vi "Handle Valve Status.vi"(10 "Response Data":T1, 11 "Control Valves in":T2) -> (3 "Control Valves out":T2)   [LabVIEW 2024, in "pumploop_client.lvlib"]
uses:
  pumploop_client/pumploop_client.lvlib
  controls/Valves--cluster.ctl
  pumploop_client/RPC Messages/pumploop_Valves.ctl
panel:
  # "Open"
  # "Closed"
  # "Open"
  # "Closed"
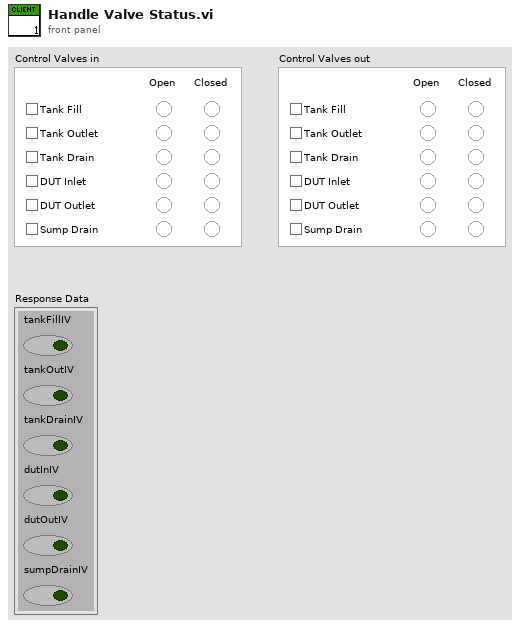
[diagram p1: front panel]
types:
  T1 = typedef "pumploop_client.lvlib/pumploop_Valves.ctl" = cluster{"tankFillIV":bool, "tankOutIV":bool, "tankDrainIV":bool, "dutInIV":bool, "dutOutIV":bool, "sumpDrainIV":bool}
  T2 = typedef "Valves--cluster.ctl" = cluster{"Tank Fill":bool, "Tank Outlet":bool, "Tank Drain":bool, "DUT Inlet":bool, "DUT Outlet":bool, "Sump Drain":bool, "Tank Fill Open":bool, "Tank Fill Closed":bool, "Tank Outlet Open":bool, "Tank Outlet Closed":bool, "Tank Drain Open":bool, "Tank Drain Closed":bool, "DUT Inlet Open":bool, "DUT Inlet Closed":bool, "DUT Outlet Open":bool, "DUT Outlet Closed":bool, "Sump Drain Open":bool, "Sump Drain Closed":bool}
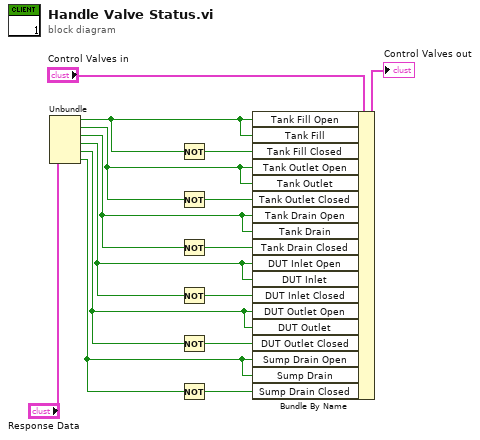
[diagram p0: block diagram]
diagram:
  n1 = Unbundle("Response Data") -> ("tankFillIV"=w6:bool, "tankOutIV"=w5:bool, "tankDrainIV"=w4:bool, "dutInIV"=w3:bool, "dutOutIV"=w2:bool, "sumpDrainIV"=w1:bool)
  n2 = Not(x=w6) -> (.not. x?=w8:bool)
  n3 = Not(x=w5) -> (.not. x?=w9:bool)
  n4 = Not(x=w4) -> (.not. x?=w10:bool)
  n5 = Not(x=w3) -> (.not. x?=w11:bool)
  n6 = Not(x=w2) -> (.not. x?=w12:bool)
  n7 = Not(x=w1) -> (.not. x?=w13:bool)
  n8 = Bundle By Name(cluster="Control Valves in", "Tank Fill Open"=w6, "Tank Fill"=w6, "Tank Fill Closed"=w8, "Tank Outlet Open"=w5, "Tank Outlet"=w5, "Tank Outlet Closed"=w9, "Tank Drain Open"=w4, "Tank Drain"=w4, "Tank Drain Closed"=w10, "DUT Inlet Open"=w3, "DUT Inlet"=w3, "DUT Inlet Closed"=w11, "DUT Outlet Open"=w2, "DUT Outlet"=w2, "DUT Outlet Closed"=w12, "Sump Drain Open"=w1, "Sump Drain"=w1, "Sump Drain Closed"=w13) -> (→"Control Valves out":T2)
